vi "Zone Dialog.vi"(10 "Rect":T2, 11 "Zone in":T1) -> (3 "Zone":T1)   [LabVIEW 2015]
uses:
  Typedef/Zone Data.ctl
panel:
  in  "Zone Name":string
  in  "OK Button":bool
  in  "Table":string[][](table)
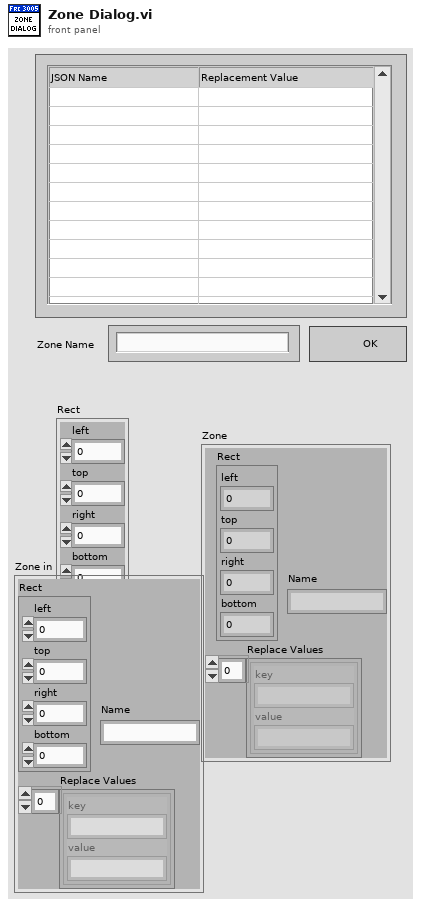
[diagram p1: front panel]
types:
  T1 = typedef "Zone Data.ctl" = cluster{"Rect":cluster{"left":i16, "top":i16, "right":i16, "bottom":i16}, "Replace Values":cluster{"key":string, "value":string}[], "Name":string}
  T2 = cluster{"left":i16, "top":i16, "right":i16, "bottom":i16}
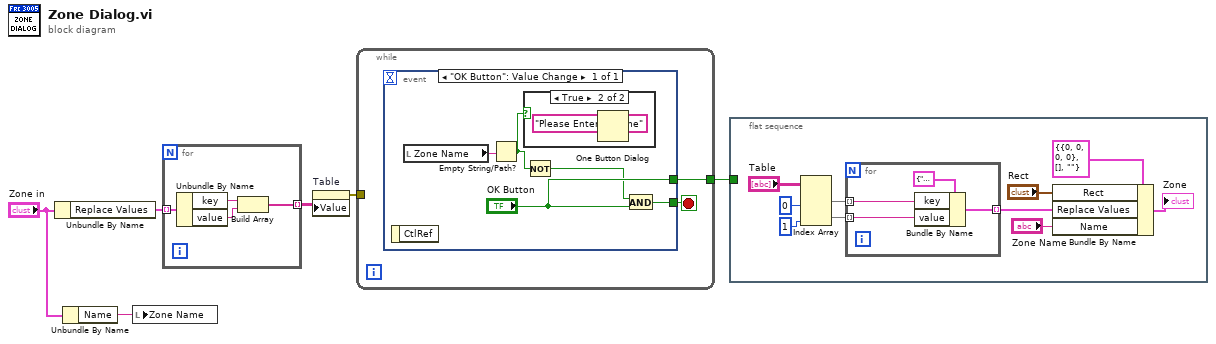
[diagram p0: block diagram]
diagram:
  n1 = Unbundle By Name("Zone in") -> ("Replace Values"=w4:cluster{"key":string, "value":string}[])
  n2 = Unbundle By Name("Zone in") -> ("Name"=w1:string)
  n3 = local write "Zone Name"(w1) -> ()
  n4 = for {
    tunnel: w4 -> [w10] mode=indexing
    tunnel: [w7] -> w3 mode=indexing
    n5 = Unbundle By Name(w10) -> ("key"=w8:string, "value"=w9:string)
    n6 = Build Array(w8, w9) -> (w7:string[])
  }
  n7 = property on="Table" class="Tbl (strict)"("Value"=w3) -> (error out=w5:errorcluster)  [unwired: 2 in, 1 out]
  n8 = while {
    tunnel: [w12] -> w6
    tunnel: w5 -> [_]
    stop <- w11 stop-if-true
    n9 = event shown="[0] \"OK Button\": Value Change" {
      selector: _ -> [_]
      dyn-events: _ -> [_]
      timeout: _ -> [_]
      tunnel: ["OK Button"] -> w12
      tunnel: [w16] -> w11
      event "OK Button": Value Change {
        n10 = event-data() -> ()  [unwired: 1 in, 1 out]
        n11 = local read "Zone Name"() -> (w15:string)
        n12 = Empty String/Path?(string/path=w15) -> (empty?=w13:bool)
        n13 = case shown="True" w13 {
          frame False {
          }
          frame True {
            n14 = One Button Dialog(message="Please Enter a Name") -> ()  [unwired: 1 in, 1 out]
          }
        }
        n15 = Not(x=w13) -> (.not. x?=w14:bool)
        n16 = And(x=w14, y="OK Button") -> (x .and. y?=w16:bool)
      }
    }
  }
  n17 = flat-sequence {
    tunnel: w6 -> [_]
    frame #0 {
      n18 = Index Array(array="Table", index (col) #1=0 ("disabled index (col)"), index (col) #2=1 ("disabled index (col)")) -> (element #1=w25:string[], element #2=w24:string[])  [unwired: 2 in]
      n19 = for {
        tunnel: w25 -> [w31] mode=indexing
        tunnel: w24 -> [w30] mode=indexing
        tunnel: [w29] -> w23 mode=indexing
        n20 = Bundle By Name(cluster=cluster{"key":string, "value":string} {"key"="", "value"=""}, "key"=w31, "value"=w30) -> (w29:cluster{"key":string, "value":string})
      }
      n21 = Bundle By Name(cluster=T1 {"Rect"={"left"=0, "top"=0, "right"=0, "bottom"=0}, "Replace Values"=[], "Name"=""}, "Rect"="Rect", "Replace Values"=w23, "Name"="Zone Name") -> (→"Zone":T1)
    }
  }
